vi "m1m3_getEvent_RejectedActiveOpticForces.vi"(8 "error in (no error)":errorcluster, 11 "logevent_RejectedActiveOpticForces_Ctl":T1) -> (0 "error out":errorcluster, 2 "function return":i32, 3 "logevent_RejectedActiveOpticForces_Ctl out":T1)   [LabVIEW 2016, in "SALLV_m1m3.lvlib"]
doc: "int m1m3_shm_getEvent_RejectedActiveOpticForcesLV(m1m3_logevent_RejectedActiveOpticForcesLV *logevent_RejectedActiveOpticForces_Ctl );"
uses:
  SALLV_m1m3.lvlib
  DataTypes/logevent_RejectedActiveOpticForces.ctl
  SALLV_m1m3.so
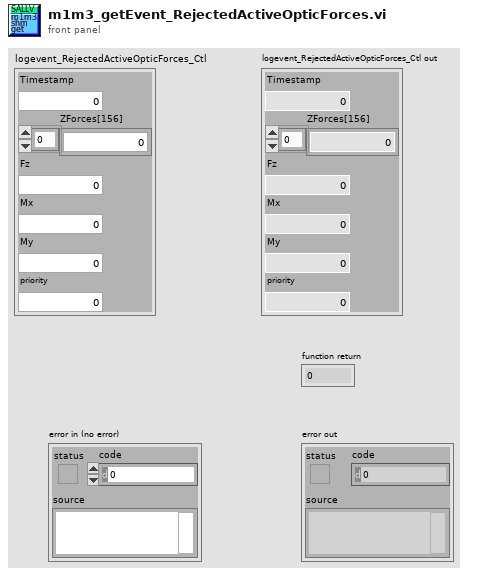
[diagram p1: front panel]
types:
  T1 = typedef "SALLV_m1m3.lvlib/logevent_RejectedActiveOpticForces.ctl" = cluster{"Timestamp":dbl, "ZForces[156]":sgl[], "Fz":sgl, "Mx":sgl, "My":sgl, "priority":i32}
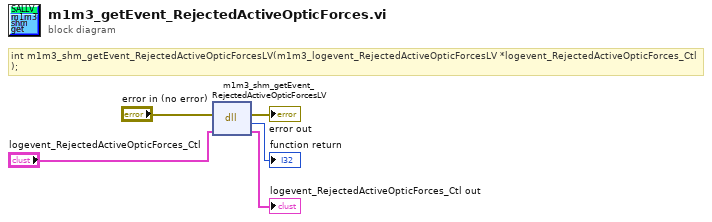
[diagram p0: block diagram]
diagram:
  # "int m1m3_shm_getEvent_RejectedActiveOpticForcesLV(m1m3_logevent_RejectedActiveOpticForcesLV *logevent_RejectedActiveOpticForces_Ctl );"
  n1 = dll-call lib="opt/CODE/SALLV_m1m3/SALLV_m1m3.*" fn="m1m3_shm_getEvent_RejectedActiveOpticForcesLV"(error in="error in (no error)", "logevent_RejectedActiveOpticForces_Ctl"="logevent_RejectedActiveOpticForces_Ctl") -> (error out=→"error out":errorcluster, →"function return":i32, "logevent_RejectedActiveOpticForces_Ctl"=→"logevent_RejectedActiveOpticForces_Ctl out":T1)  [unwired: 2 in, 1 out]
